vi "isVerbose.vi"(11 "Assert in":refnum<class "Assert.lvclass">) -> (2 "Verbose":bool, 3 "Assert out":refnum<class "Assert.lvclass">)   [LabVIEW 2013, in "Caraya.lvlib" / "Assert.lvclass"]
uses:
  Assert.lvclass
  Assert.lvclass/Assert.ctl
  Basic Test Manager/Basic Test Manager.lvclass/Basic Test Manager.ctl
  Basic Test Manager/Basic Test Manager.lvclass
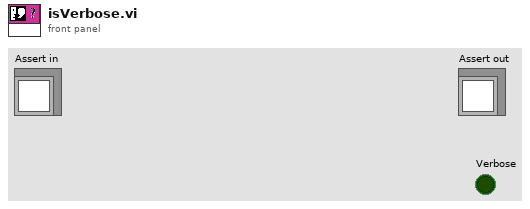
[diagram p1: front panel]
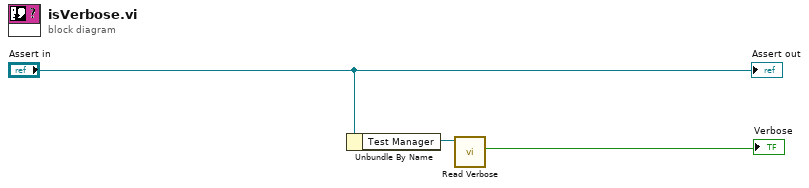
[diagram p0: block diagram]
diagram:
  n1 = Unbundle By Name("Assert in") -> ("Test Manager"=w3:refnum<class "Basic Test Manager.lvclass">)
  n2 = call "Read Verbose.vi"("Basic Test Manager"=w3) -> ("Verbose"=→"Verbose":bool)  [unwired: 8 in, 2 out]
  "Assert out" <- "Assert in"
